vi "midi_GetBytes.vi"(8 "error in (no error)":errorcluster, 11 "folder name":path) -> (0 "error out":errorcluster, 2 "length":i64, 3 "string":string)   [LabVIEW 2013]
doc: "Read contents of a file and return as a string. The number of bytes read is also available."
panel:
  # "midi_GetBytes"
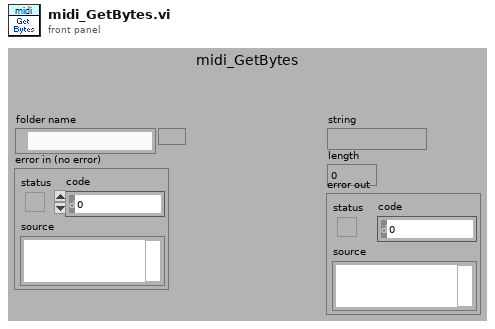
[diagram p1: front panel]
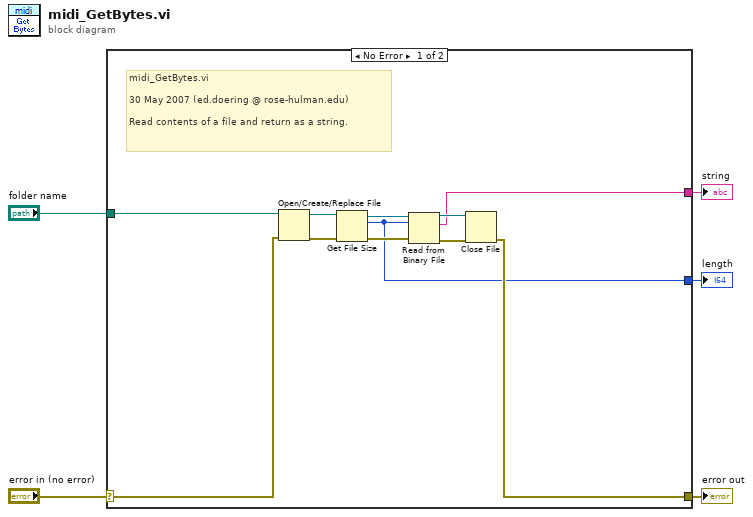
[diagram p0: block diagram]
diagram:
  n1 = case shown="No Error" "error in (no error)" {
    selector: "error in (no error)" -> [w10 w17]
    tunnel: [w8 w17] -> w1
    tunnel: "folder name" -> [w6 _]
    tunnel: [w9 _] -> w3
    tunnel: [w7 _] -> w2
    frame No Error {
      # "midi_GetBytes.vi\n\n30 May 2007 (ed.doering @ rose-hulman.edu)\n\nRead contents of a file and return as a string."
      n2 = Open/Create/Replace File(file path (use dialog)=w6, error in=w10) -> (refnum out=w16:refnum<file>, error out=w15:errorcluster)  [unwired: 4 in, 1 out]
      n3 = Get File Size(file=w16, error in=w15) -> (refnum out=w14:refnum<file>, size (in bytes)=w7:i64, 0:w13:errorcluster)
      n4 = Read from Binary File(8:w13, 10:w7, 11:w14) -> (0:w12:errorcluster, 2:w9:string, 3:w11:refnum<file>)  [unwired: 3 in, 1 out]
      n5 = Close File(refnum=w11, error in=w12) -> (error out=w8:errorcluster)  [unwired: 1 out]
    }
    frame Error {
    }
  }
  "string" <- w3
  "length" <- w2
  "error out" <- w1
